vi "LJLogM read channels.vi"(0 "Handle In":i32, 5 "# Channels":i32, 9 "Channel Setup In":T1={"Name"=["AIN0", "AIN1", "AIN2", "AIN3", "AIN4", "AIN5", "AIN6", "AIN7", "AIN8", "AIN9", "AIN10", "AIN11", "AIN12", "AIN13", "AIN14", "AIN15"], "", "Scaling Equation"=["y=a", "y=b", "y=c", "y=d", "y=e", "y=f", "y=g", "y=h", "y=i", "y=j", "y=k", "y=l", "y=m", "y=n", "y=o", "y=p"], "", "Graph?"=[TRUE, TRUE, TRUE, TRUE, FALSE, FALSE, FALSE, FALSE, FALSE, FALSE, FALSE, FALSE, FALSE, FALSE, FALSE, FALSE]}, 11 "Error In":errorcluster) -> (3 "Timestamp":timestamp, 4 "Handle Out":i32, 6 "Raw Data":dbl[](array[numeric]), 8 "Scaled Data":dbl[](array[numeric]), 12 "Error Message":string="No Error", 14 "Error Message Status":bool, 15 "(LJM) Error Out":errorcluster)   [LabVIEW 2026]
uses:
  Common Logger Controls/Channel Setup.ctl
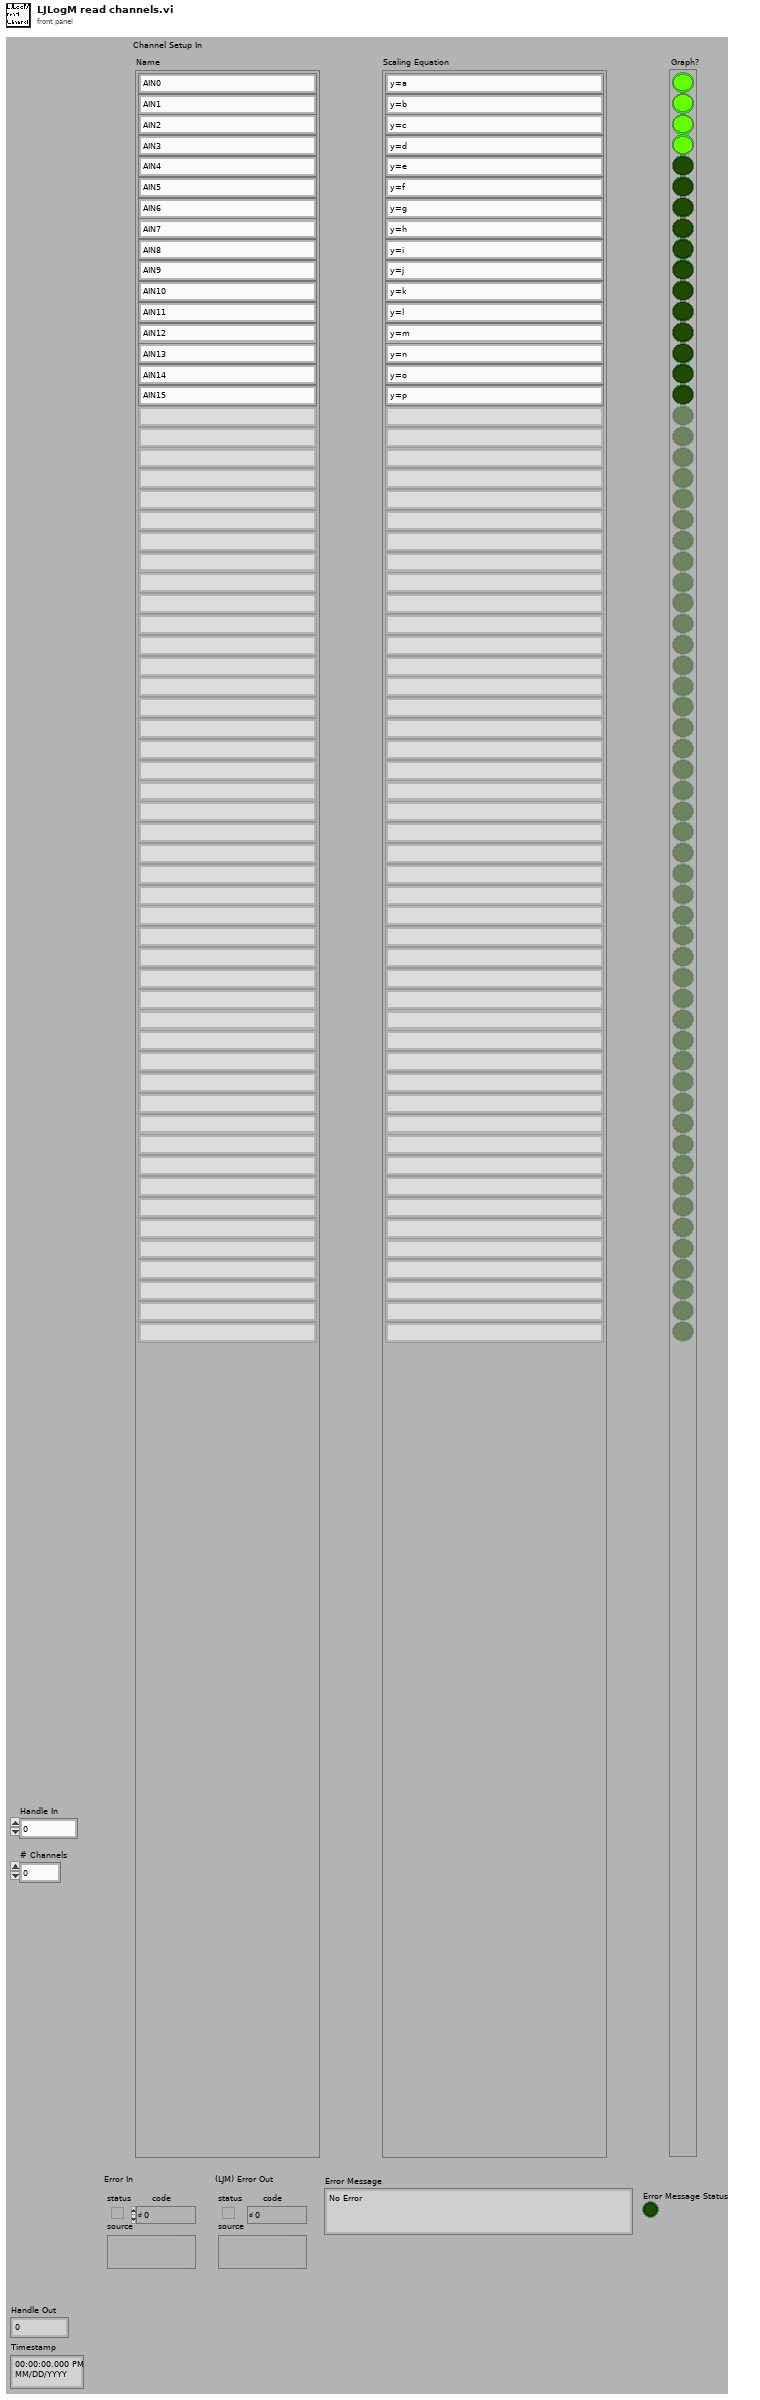
[diagram p1: front panel]
types:
  T1 = typedef "Channel Setup.ctl" = cluster{"Name":string[], string, "Scaling Equation":string[], string, "Graph?":bool[]}
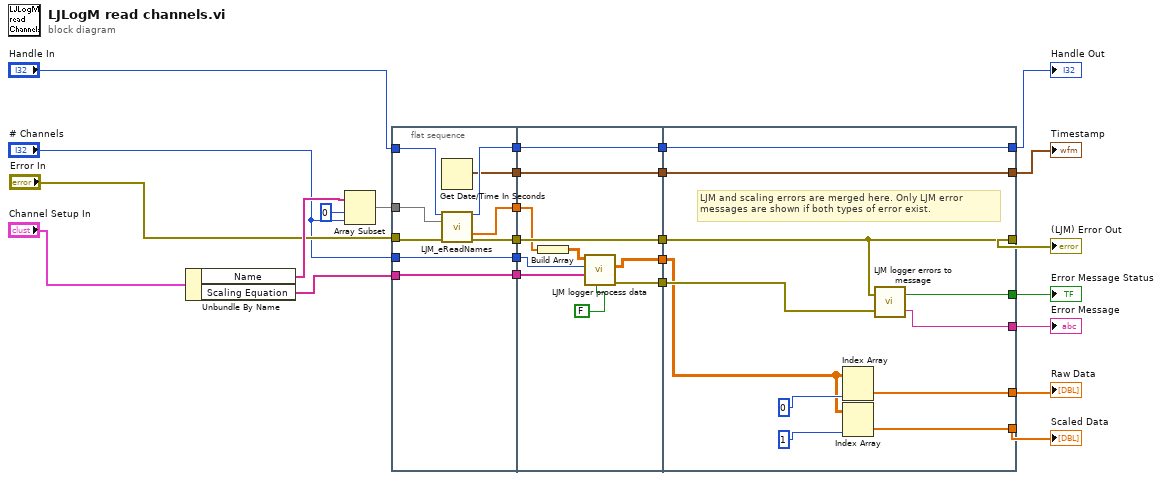
[diagram p0: block diagram]
diagram:
  n1 = Unbundle By Name("Channel Setup In") -> ("Name"=w24:string[], "Scaling Equation"=w12:string[])
  n2 = Array Subset(array=w24, index=0 ("Array Index"), length="# Channels") -> (w25:string[])
  n3 = flat-sequence {
    tunnel: w25 -> [w35]
    tunnel: "Error In" -> [w33]
    tunnel: "Handle In" -> [w32]
    tunnel: [w34] -> w20
    tunnel: [w31] -> w19
    tunnel: [w30] -> w18
    tunnel: w12 -> [w29]
    tunnel: [w29] -> w13
    tunnel: [w28] -> w8
    tunnel: "# Channels" -> [w28]
    tunnel: [w27] -> w1
    tunnel: w20 -> [w37]
    tunnel: w19 -> [w45]
    tunnel: w18 -> [w44]
    tunnel: [w45] -> w16
    tunnel: [w44] -> w15
    tunnel: [w36] -> w14
    tunnel: w13 -> [w40]
    tunnel: w8 -> [w39]
    tunnel: [w43] -> w3
    tunnel: [w42] -> w2
    tunnel: w1 -> [w36]
    tunnel: [w55] -> w17
    tunnel: [w50] -> w9
    tunnel: [w56] -> w21
    tunnel: w16 -> [w56]
    tunnel: w15 -> [w50]
    tunnel: w14 -> [w55]
    tunnel: [w52] -> w11
    tunnel: [w51] -> w10
    tunnel: [w49] -> w5
    tunnel: [w48] -> w4
    tunnel: w3 -> [w47]
    tunnel: w2 -> [w46]
    frame #0 {
      n4 = Get Date/Time In Seconds() -> (seconds since 1Jan1904=w27:timestamp)
      n5 = call "LJM_eReadNames.vi"("Handle In"=w32, "aNames"=w35, "error in"=w33) -> ("Handle Out"=w31:i32, "aValuesOut"=w34:dbl[], "error out"=w30:errorcluster)  [unwired: 9 in, 1 out]
    }
    frame #1 {
      n6 = Build Array(w37) -> (w38:dbl[][])
      n7 = call "LJM logger process data.vi"("Disable Scaling"=FALSE, "Scaling Equation"=w40, "# Channels"=w39, "Voltages"=w38) -> ("error out"=w43:errorcluster, "Volts,Scaled Averages"=w42:dbl[][])  [unwired: 5 in, 1 out]
    }
    frame #2 {
      # "LJM and scaling errors are merged here. Only LJM error messages are shown if both types of error exist."
      n8 = Index Array(array=w46, index (col)=0 ("Disabled Index (col)")) -> (element=w49:dbl[])  [unwired: 1 in]
      n9 = Index Array(array=w46, index (col)=1 ("Disabled Index (col)")) -> (element=w48:dbl[])  [unwired: 1 in]
      n10 = call "LJM logger errors to message.vi"("Scaling Error"=w47, "LJM Error"=w50) -> ("Error Message"=w51:string, "status"=w52:bool)
    }
  }
  "Handle Out" <- w21
  "Timestamp" <- w17
  "(LJM) Error Out" <- w9
  "Error Message" <- w10
  "Error Message Status" <- w11
  "Raw Data" <- w5
  "Scaled Data" <- w4
